vi "Handle Command.vi"(8 "error in":errorcluster, 10 "CMD in":refnum<class "Update Red DC.lvclass">, 11 "Object In":refnum<class>) -> (0 "error out":errorcluster, 1 "Command Successful?":bool, 2 "CMD out":refnum<class "Update Red DC.lvclass">, 3 "Object Out":refnum<class>)   [LabVIEW 2014, in "eCRDS Library.lvlib" / "Update Red DC.lvclass"]
doc: "This VI will contain the code used to actually execute the request. If the request is successful, this will be indicated by the boolean output <b>Command Successful?</b>. The boolean output can then be used by the <b>Command Reply</b> which sends a reply if the reply queue is valid."
uses:
  Update Red DC.lvclass
  Main/eCRDS.lvclass
  <vilib>/DAQmx/configure/timing.llb/DAQmx Timing (Implicit).vi
  <resource>/objmgr/daqmx.rc
  reusable/Session APIs/Session Log/System Log.lvclass
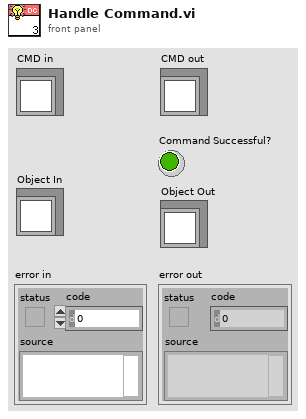
[diagram p1: front panel]
types:
  T1 = typedef "Session - Root.lvclass/Session Handle.ctl" = refnum<data-value>
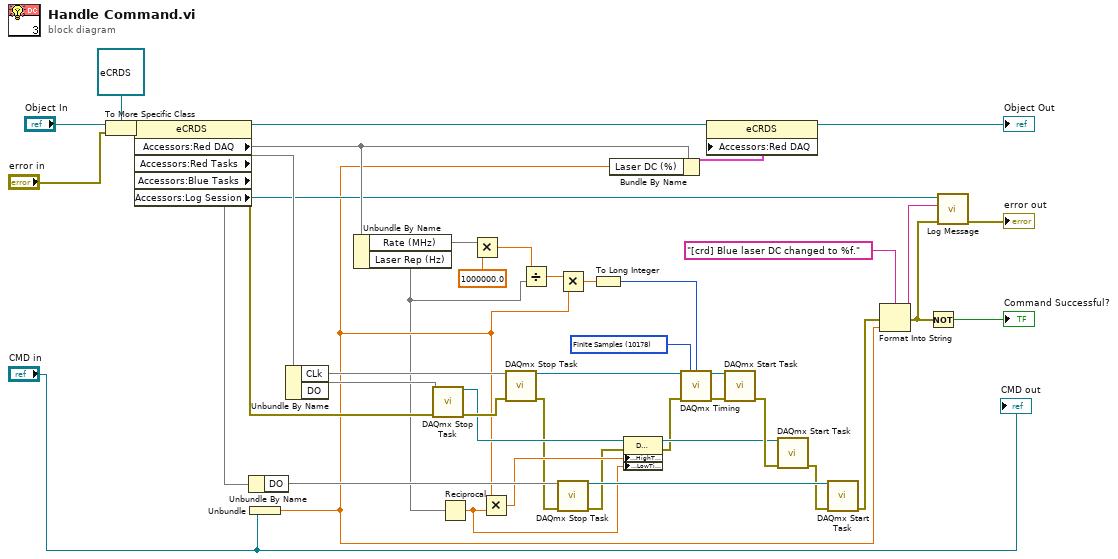
[diagram p0: block diagram]
diagram:
  w31 = 10178 items=["Finite Samples"=10178, "Continuous Samples"=10123, "Hardware Timed Single Point"=12522] ("sample mode")
  n1 = To More Specific Class(target class=refnum<class "eCRDS.lvclass"> refnum ("eCRDS"), reference="Object In", error in="error in") -> (specific class reference=w39:refnum<class "eCRDS.lvclass">, error out=w37:errorcluster)
  n2 = property class="eCRDS"(reference=w39, error in=w37) -> (reference out=w17:refnum<class "eCRDS.lvclass">, error out=w19:errorcluster, "Accessors:Red DAQ"=w38, "Accessors:Red Tasks"=w36, "Accessors:Blue Tasks"=w35, "Accessors:Log Session"=w12:T1)
  n3 = Unbundle By Name(w35) -> ("DO"=w33)
  n4 = Unbundle("CMD in") -> (w2:dbl)
  n5 = Unbundle By Name(w36) -> ("CLk"=w32, "DO"=w34)
  n6 = Unbundle By Name(w38) -> ("Rate (MHz)"=w29, "Laser Rep (Hz)"=w1)
  n7 = call <vilib>:"DAQmx Stop Task.vi"("task/channels in"=w34, "error in"=w19) -> ("task out"=w15:refnum<k21>, "error out"=w18:errorcluster)  [unwired: 12 in]
  n8 = Reciprocal(x=w1) -> (1/x=w7:dbl)
  n9 = Multiply(x=w29, y=1000000.0) -> (x*y=w27:dbl)
  n10 = Multiply(x=w2, y=w7) -> (x*y=w8:dbl)
  n11 = call <vilib>:"DAQmx Stop Task.vi"("task/channels in"=w32, "error in"=w18) -> ("task out"=w30:refnum<k21>, "error out"=w6:errorcluster)  [unwired: 12 in]
  n12 = Divide(x=w27, y=w1) -> (x/y=w26:dbl)
  n13 = Multiply(x=w26, y=w2) -> (x*y=w25:dbl)
  n14 = call <vilib>:"DAQmx Stop Task.vi"("task/channels in"=w33, "error in"=w6) -> ("task out"=w20:refnum<k21>, "error out"=w5:errorcluster)  [unwired: 12 in]
  n15 = To Long Integer(number=w25) -> (32bit integer=w24:i32)
  n16 = Bundle By Name(cluster=w38, "Laser DC (%)"=w2) -> (w16:cluster{})
  n17 = property class="DAQmx Channel"(reference=w15, error in=w5, "CO.Pulse.HighTime"=w8, "CO.Pulse.LowTime"=w7) -> (reference out=w14:refnum<k21>, error out=w13:errorcluster)
  n18 = call-poly <vilib>:"DAQmx Timing.vi"("task/channels in"=w30, "sample mode"=w31, "samples per channel"=w24, "error in"=w13) -> ("task out"=w23:refnum<k21>, "error out"=w22:errorcluster)  [unwired: 10 in]
  n19 = property class="eCRDS"(reference=w17, "Accessors:Red DAQ"=w16) -> (reference out=→"Object Out":refnum<class "eCRDS.lvclass">)  [unwired: 1 in, 1 out]
  n20 = call <vilib>:"DAQmx Start Task.vi"("task/channels in"=w23, "error in"=w22) -> ("error out"=w21:errorcluster)  [unwired: 12 in, 1 out]
  n21 = call <vilib>:"DAQmx Start Task.vi"("task/channels in"=w14, "error in"=w21) -> ("error out"=w4:errorcluster)  [unwired: 12 in, 1 out]
  n22 = call <vilib>:"DAQmx Start Task.vi"("task/channels in"=w20, "error in"=w4) -> ("error out"=w3:errorcluster)  [unwired: 12 in, 1 out]
  n23 = Format Into String(format string="[crd] Blue laser DC changed to %f.", error in=w3, w2) -> (resulting string=w10:string, error out=w9:errorcluster)  [unwired: 1 in]
  n24 = Not(x=w9) -> (.not. x?=→"Command Successful?":bool)
  n25 = call "Log Message.vi"("error in"=w9, "MSG In"=w10, "session in"=w12) -> ("error out"=→"error out":errorcluster)  [unwired: 7 in, 1 out]
  "CMD out" <- "CMD in"
